vi "UtilityLib.TCPNoDelay.vi"(8 "error in (no error)":errorcluster, 10 "no delay (on)":bool=TRUE, 11 "connection in":refnum<k5>) -> (0 "error out":errorcluster, 3 "connection out":refnum<k5>)   [LabVIEW 2014, in "UtilityLib.lvlib"]
doc: "Turn TCP_NODELAY on or off on the given network refnum.\n\nNOTE: This calls Windows95/NT specific functions and will only work on those platforms.."
uses:
  UtilityLib.lvlib
  wsock32.dll
  lib/libc-2.10.1.so
panel:
  out "setsockopt result":i32
  # "Turn TCP_NODELAY on or off on the given network refnum."
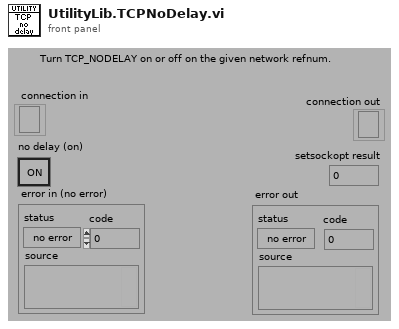
[diagram p1: front panel]
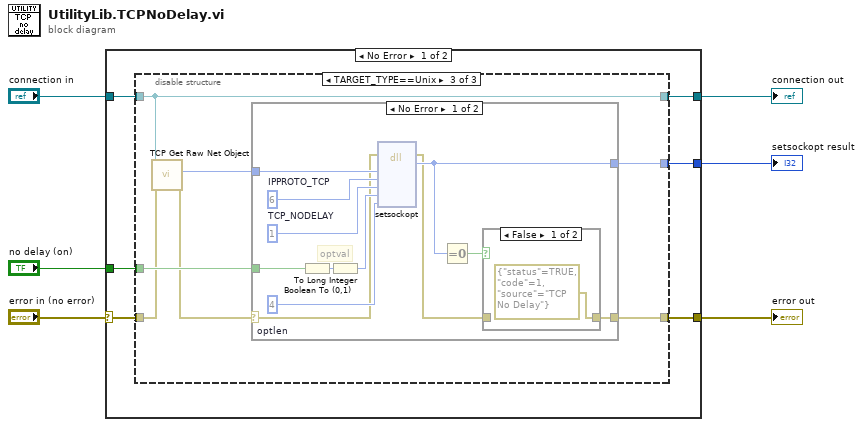
[diagram p0: block diagram]
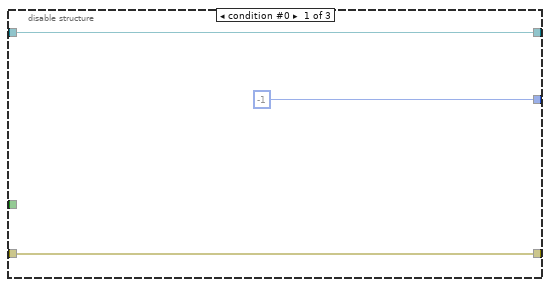
[diagram p2: hidden frame]
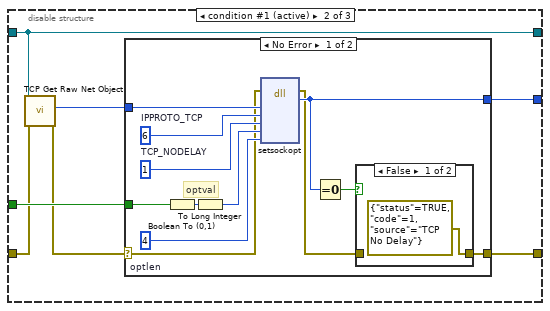
[diagram p3: hidden frame]
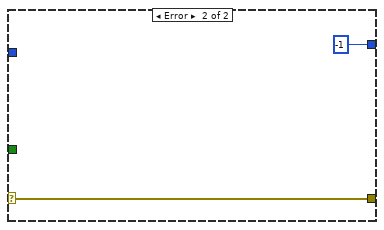
[diagram p5: hidden frame]
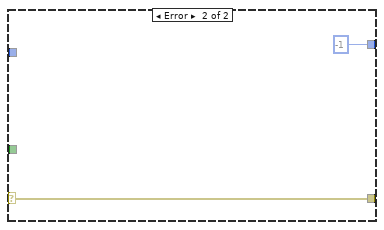
[diagram p7: hidden frame]
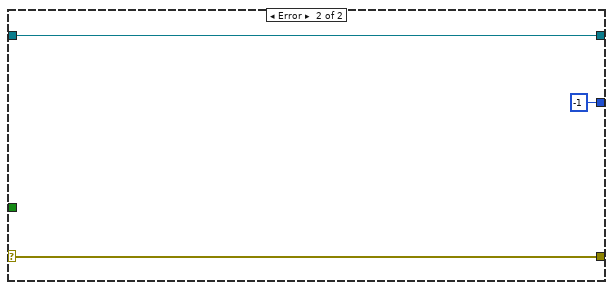
[diagram p8: hidden frame]
diagram:
  n1 = case shown="No Error" "error in (no error)" {
    selector: "error in (no error)" -> [w10 w64]
    tunnel: "connection in" -> [w12 w63]
    tunnel: "no delay (on)" -> [w8 _]
    tunnel: [w9 w64] -> w3
    tunnel: [w11 w63] -> w2
    tunnel: [w7 -1 ("return value")] -> w1
    frame No Error {
      n2 = disable-structure shown="TARGET_TYPE==Unix" {
        disable-tunnel: [w15 w21 w44] -> w11
        disable-tunnel: w12 -> [w15 w21 w44]
        disable-tunnel: [w14 w17 w40] -> w9
        disable-tunnel: w10 -> [w14 w19 w42]
        disable-tunnel: w8 -> [_ w20 w43]
        disable-tunnel: [-1 ("return value") w16 w39] -> w7
        frame condition #0 {
        }
        frame condition #1 (active) {
          n3 = call <vilib>:"TCP Get Raw Net Object.vi"("error in (no error)"=w19, "connection ID"=w21) -> ("error out"=w18:errorcluster, "raw net object"=w22:u64)  [unwired: 7 in, 1 out]
          n4 = case shown="No Error" w18 {
            selector: w18 -> [w24 w37]
            tunnel: [w26 w37] -> w17
            tunnel: w22 -> [w34 _]
            tunnel: [w28 -1] -> w16
            tunnel: w20 -> [w25 _]
            frame No Error {
              w29 = 1  # TCP_NODELAY
              w30 = 6  # IPPROTO_TCP
              w33 = 4  # optlen
              # "optval"
              n5 = Boolean To (0,1)(Boolean=w25) -> (0, 1=w32:i16)
              n6 = To Long Integer(number=w32) -> (32bit integer=w31:i32)
              n7 = dll-call lib="wsock32.dll" fn="setsockopt"(error in=w24, "s"=w34, "level"=w30, "optname"=w29, "optval"=w31, "optlen"=w33) -> (error out=w23:errorcluster, "return value"=w28:i32)  [unwired: 7 in, 1 out]
              n8 = Equal To 0?(x=w28) -> (x = 0?=w27:bool)
              n9 = case shown="False" w27 {
                tunnel: w23 -> [_ w36]
                tunnel: [errorcluster {"status"=TRUE, "code"=1, "source"="TCP No Delay"} ("error in (no error)") w36] -> w26
                frame False {
                }
                frame True {
                }
              }
            }
            frame Error {
            }
          }
        }
        frame condition #2 {
          n10 = call <vilib>:"TCP Get Raw Net Object.vi"("error in (no error)"=w42, "connection ID"=w44) -> ("error out"=w41:errorcluster, "raw net object"=w45:u64)  [unwired: 7 in, 1 out]
          n11 = case shown="No Error" w41 {
            selector: w41 -> [w47 w60]
            tunnel: [w49 w60] -> w40
            tunnel: w45 -> [w57 _]
            tunnel: [w51 -1] -> w39
            tunnel: w43 -> [w48 _]
            frame No Error {
              w52 = 1  # TCP_NODELAY
              w53 = 6  # IPPROTO_TCP
              w56 = 4  # optlen
              # "optval"
              n12 = Boolean To (0,1)(Boolean=w48) -> (0, 1=w55:i16)
              n13 = To Long Integer(number=w55) -> (32bit integer=w54:i32)
              n14 = dll-call lib="lib/libc-2.10.1.so" fn="setsockopt"(error in=w47, "s"=w57, "level"=w53, "optname"=w52, "optval"=w54, "optlen"=w56) -> (error out=w46:errorcluster, "return value"=w51:i32)  [unwired: 7 in, 1 out]
              n15 = Equal To 0?(x=w51) -> (x = 0?=w50:bool)
              n16 = case shown="False" w50 {
                tunnel: w46 -> [_ w59]
                tunnel: [errorcluster {"status"=TRUE, "code"=1, "source"="TCP No Delay"} ("error in (no error)") w59] -> w49
                frame False {
                }
                frame True {
                }
              }
            }
            frame Error {
            }
          }
        }
      }
    }
    frame Error {
    }
  }
  "connection out" <- w2
  "error out" <- w3
  "setsockopt result" <- w1
